vi "Example Simple.vi"() -> ()   [LabVIEW 2013]
uses:
  C:/tf/play/labview/Tinkerforge.dll
  Tinkerforge.dll
panel:
  out "voltage (V)":sgl
  in  "uid":string="amb"
  in  "port":i32=4223
  in  "host":string="localhost"
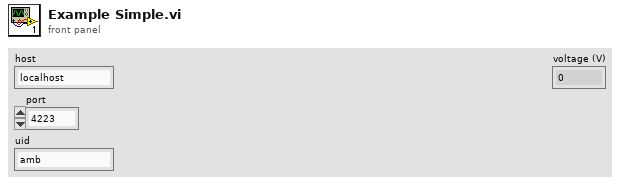
[diagram p1: front panel]
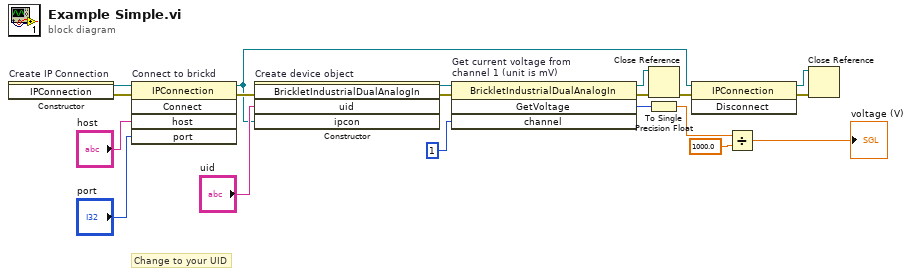
[diagram p0: block diagram]
diagram:
  # "Change to your UID"
  n1 = constructor on="Create IP Connection" class="IPConnection"() -> (reference out=w19:refnum<k24>, error out=w2:errorcluster)  [unwired: 3 in, 1 out]
  n2 = invoke on="Connect to brickd" class="IPConnection" method="Connect"(reference=w19, error in=w2, "host"="host", "port"="port") -> (reference out=w8:refnum<k24>, error out=w15:errorcluster)  [unwired: 1 in, 3 out]
  n3 = constructor on="Create device object" class="BrickletIndustrialDualAnalogIn"(error in=w15, "uid"="uid", "ipcon"=w8) -> (reference out=w13:refnum<k24>, error out=w14:errorcluster)  [unwired: 2 in, 3 out]
  n4 = invoke on="Get current voltage from\nchannel 1 (unit is mV)" class="BrickletIndustrialDualAnalogIn" method="GetVoltage"(reference=w13, error in=w14, "channel"=u8 1 ("sensor")) -> (reference out=w11:refnum<k24>, error out=w12:errorcluster, "GetVoltage"=w6:i32)  [unwired: 1 in, 1 out]
  n5 = Close Reference(reference=w11, error in (no error)=w12) -> (error out=w10:errorcluster)
  n6 = To Single Precision Float(number=w6) -> (single precision float=w4:sgl)
  n7 = invoke class="IPConnection" method="Disconnect"(reference=w8, error in=w10) -> (reference out=w7:refnum<k24>, error out=w9:errorcluster)  [unwired: 1 in, 1 out]
  n8 = Divide(x=w4, y=sgl 1000.0) -> (x/y=→"voltage (V)":sgl)
  n9 = Close Reference(reference=w7, error in (no error)=w9) -> ()  [unwired: 1 out]
